vi "WPI_DMAWordsPerEnableConstant.vi"() -> (0 "WordsPerEnable":i32[](array[numeric]))   [LabVIEW 2017]
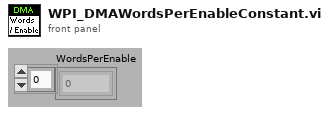
[diagram p1: front panel]
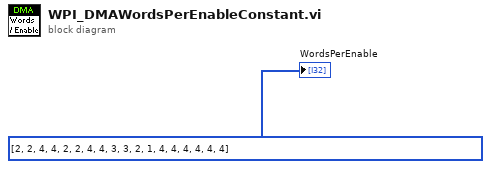
[diagram p0: block diagram]
diagram:
  "WordsPerEnable" <- i32[] [2, 2, 4, 4, 2, 2, 4, 4, 3, 3, 2, 1, 4, 4, 4, 4, 4, 4]
